vi "Testing Mode.vi"(8 "Filepath":path=path "D:/My Project/2019-2020/Magnetic Mareli UM/MM_UM/Project Setup/data/program seq/Program_280A.bin") -> (4 "Running Model":string)   [LabVIEW 2020]
uses:
  Control Button/Exit.ctl
  Control Button/Start.ctl
  Test  enqueue/AutoTest seq.ctl
  Test  enqueue/Auot Test selection.ctl
  Galobal variable_TI.vi
  Project Setup/Globle Variable/GR_Servo.vi
  <vilib>/Utility/file.llb/Read Delimited Spreadsheet (string).vi
  <vilib>/Utility/file.llb/Write Delimited Spreadsheet (string).vi
panel:
  out "Lc":dbl
  in  "Boolean":bool=TRUE
  in  "String":string
  out "Camera NG":bool
  out "Camera Ok":bool
  out "CO-ORDINATE":T1
  out "Reset":bool
  out "Emergency":bool
  out "Max Load(N)":string
  out "Min Load(N)":string
  in  "Actual Load(N)":string
  out "PPH Max(mm)":string
  out "PPH Min(mm)":string
  out "PPH(mm)":string
  out "Load Cell":dbl format="%0.03f"
  in  "Load Offset":dbl
  out "TFT Code":string
  out "Difus.Code":string
  out "max value":dbl
  out "Difusser Barcode":string
  out "Camera NG_":bool
  out "Camera OK_":bool
  out "Difusser_AI5":bool
  out "Difusser_AI4":bool
  out "Job ID":string
  in  "Graph Reset":bool
  in  "Safety Enb":bool
  in  "LCD Servo Call":bool
  out "Home":bool
  out "Start":bool
  in  "Tab Control":enum32{"Test", "Home call"}(tab)
  in  "test":string[][](table)=[["1", "Light Box Ionization", "Pass"], ["2", "Light box Clamp", "Pass"], ["3", "Difusser Put on Light Box", "Pass"], ["4", "Photo Prism Put On LB", "Test In Progress"], ["5", "LCD Put On Light Box", ""], ["6", "Difusser Checking Position", ""], ["7", "Adesive Tap check Camera", ""], ["8", "LCD Placing Position", ""], ["9", "Camera check Adhesive Taps", ""], ["10", "LCD Display Rotating ", ""], ["11", "Camera Slide Unit", ""], ["12", "LCD Pressing Servo", ""], ["13", "LCD Pressing servo up", ""], ["14", "Camera Unit Rev", ""], ["15", "Fixture Slide Up", ""], ["16", "Light Box Unclamp", ""]]
  in  "Home":string[][](table)
  out "stripped path":path
  in  "Tab":enum32{"Image Display", "Load Graph"}(tab)
  out "2D Picture":picture
  out "Boolean 3":bool
  out "Force Vs Time":dbl[](graph)
  in  "Vacuum bit":bool
  in  "LCD Servo Reset 2":bool
  out "LCD Barcode":string
  out "Date time":string
  in  "NG Counter":string
  in  "OK Counter":string
  out "User Name":string
  out "Error":bool
  in  "Cycle":i32
  in  "Slide Servo Home Call":bool
  out "D-enqueue":T2
  in  "Home Call":bool
  out "DI":bool[](array[boolean])
  in  "Error Message":string
  out "Current Date & Time":timestamp
  out "Cycle Time(Sec)":i32
  in  "Start":T3
  in  "Cycle Start Bit":bool
  in  "vi reference":refnum<vi>
  in  "Reset Ct.":bool
  out "error out":errorcluster
  in  "Tbl Refnum":refnum<vi>
  in  "Image Display":bool
  in  "Exit":T4
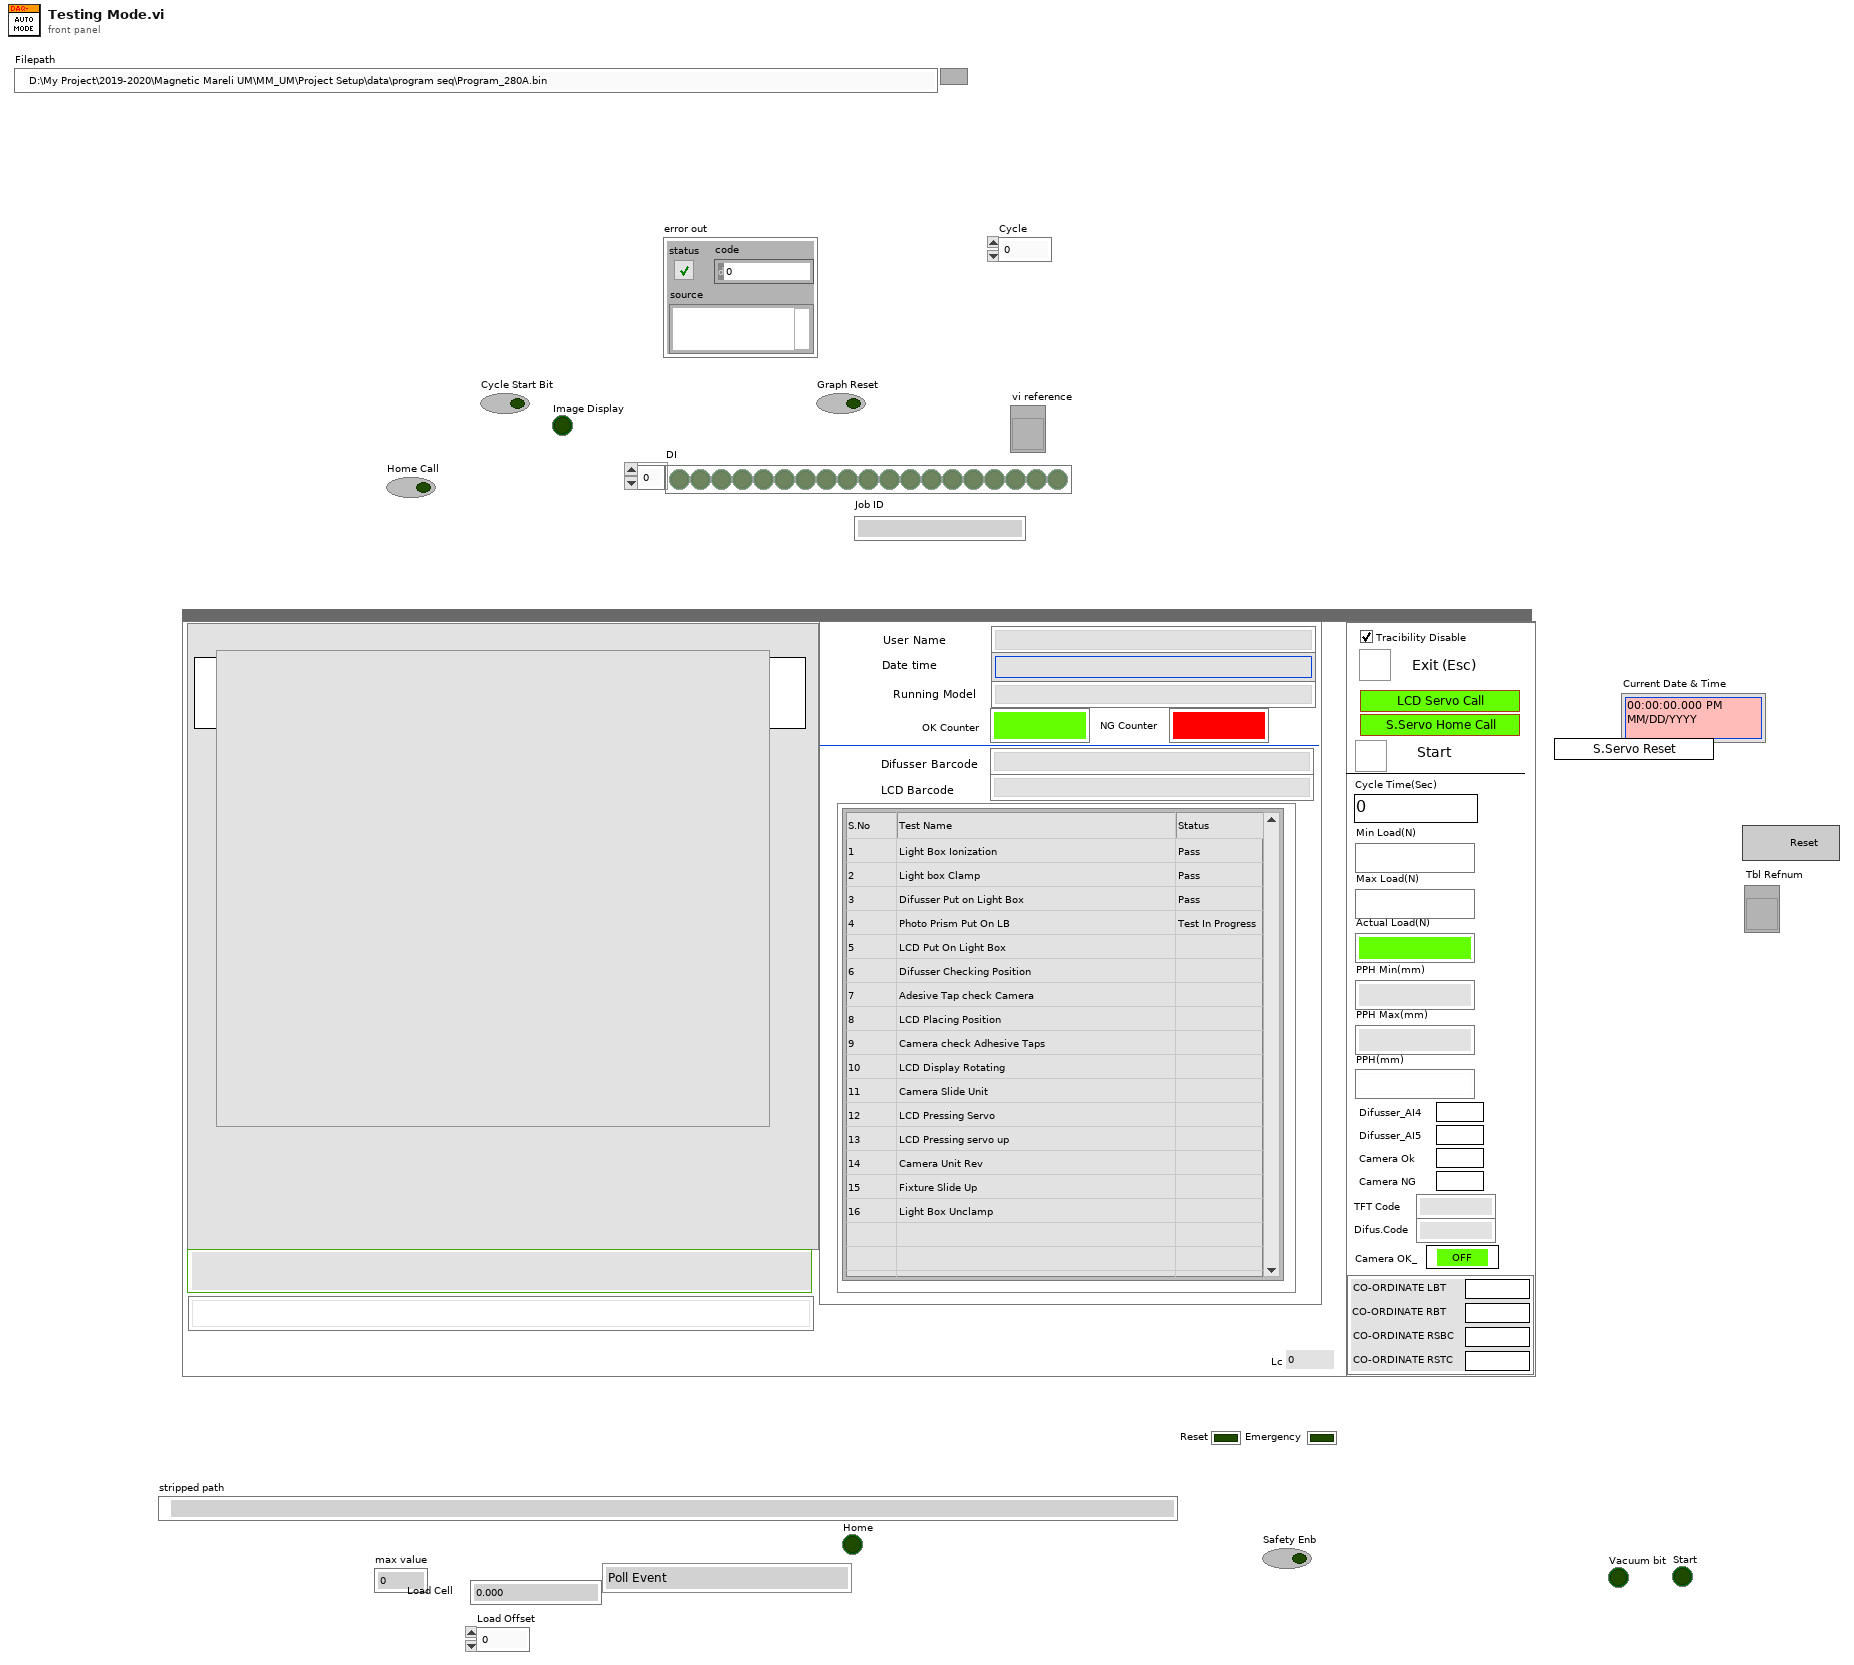
[diagram p1: front panel]
types:
  T1 = cluster{"CO-ORDINATE LBT":string, "CO-ORDINATE RBT":string, "CO-ORDINATE RSBC":string, "CO-ORDINATE RSTC":string}
  T2 = typedef "AutoTest seq.ctl" = enum16{"Poll Event", "Cylender Home ", "Initilization", "Read Barcode", "Slide Servo send Cammand", "Slide Servo Home Call", "LCD Press Servo send Cammand", "LCD Press Servo  Home Call", "Camera Co-ordinate_1", "Home Call", "Result Save", "Exit"}
  T3 = typedef "Start.ctl" = bool
  T4 = typedef "Exit.ctl" = bool
  T5 = typedef "Auot Test selection.ctl" = enum16{"Init", "Enqueue ", "Enqueue N", "Enqueue in stack", "Enqueue in stack N", "Dequeue", "Dequeue N", "Flush", "Release Queue"}
  T6 = cluster{"MaxLoad ":dbl, "Min Load":dbl, "MaxDistance(mm)":dbl, "Min Distance(mm)":dbl, "Load Offset":dbl, "Model":string, "Difusser Code":string, "TFT Code ":string, "LVDT Offset":dbl}
  T7 = cluster{"Item Name":string, "Item Status":bool, "Steps":cluster{"Channel Type":string, "Channels":string, "Wait/Poll (ms)":u32, "Parameter":u8, "STM-Speed":i32, "STM-Degree":u32, "Direction":u8}[]}[]
  T8 = cluster{"No. Fail Coun t":string, "Rework Status Count 0\\1":string, "NA Count Max =3 ":string, "Testesd Count  0/1":string, "Error code":string}
  T9 = enum16{"Height Check Cyl up(P0.23_07)", "Height Check Cyl  Up RS_(AI12_26)", "Height Check Cyl  Dn RS_(AI13_27)", "Height Check Cyl dn(P0.24_08)", "Camera Cyl Rev(P0.26_10)", "Camera Cyl fwd(P0.25_09)", "Height Check Cyl off", "Camera Cyl Rev_RS(AI15_29)", "Camera Cyl off", "Camera Cyl FWD_RS(AI14_28)", "LCD Rotation Dn(P0.28_12)", "LCD Rotation dn proxi(AI17_31)", "LCD Rotation Up(P0.27_11)", "LCD Rotation dn proxi(AI16_30)"}
  T10 = cluster{"Start":bool, "Emergency ":bool, "Reset":bool, "Home":bool, "Safety":bool}
  T11 = cluster{"[0]":string, "[1]":string, "[2]":string, "[3]":string, "[4]":string, "[5]":string, "[6]":string, "[7]":string}
  T12 = cluster{"[0]":string, "[1]":string, "[2]":string, "[3]":string, "[4]":string}
  T13 = cluster{"Emergency":bool, "Air Pressure":bool, "Saftey Sensor":bool, "Slide Servo  fault":bool, "LCD Pressing  Servo  fault":bool, "Reset":bool}
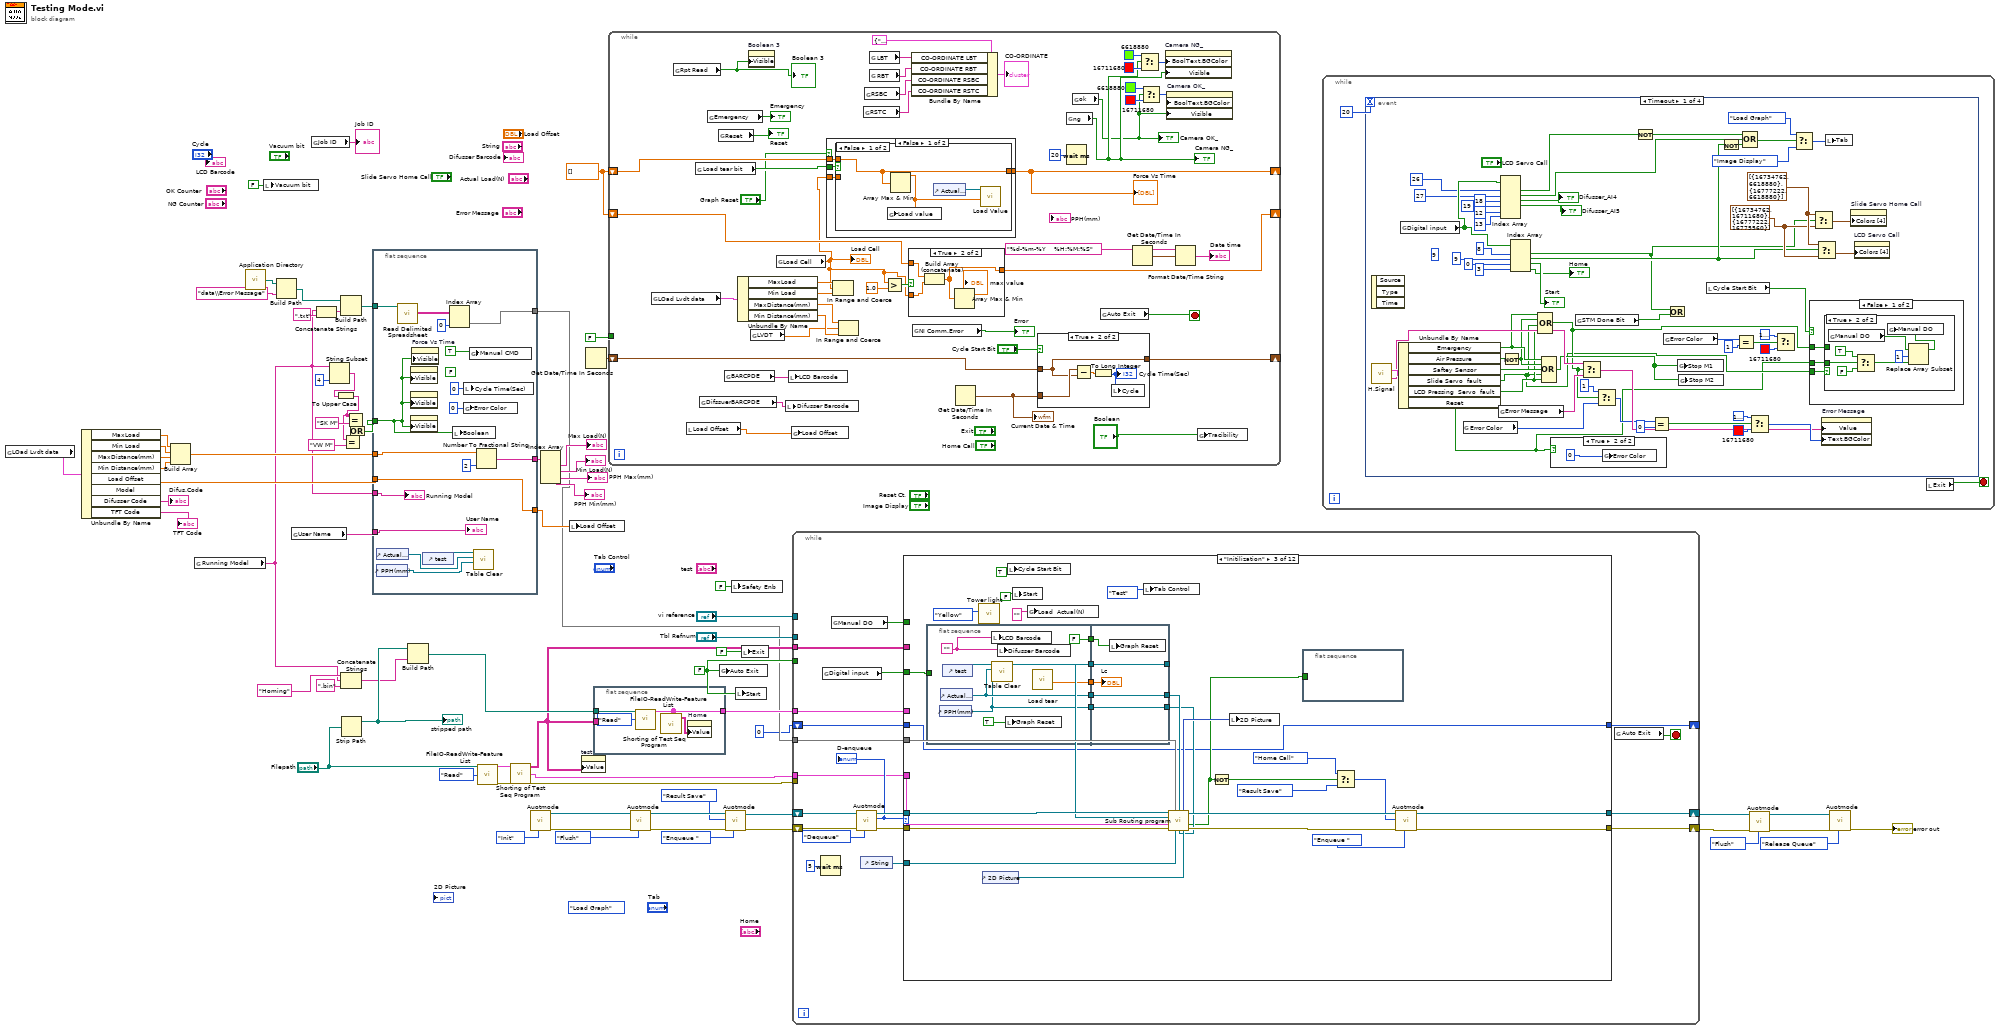
[diagram p0: block diagram]
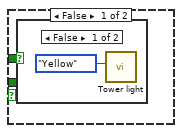
[diagram p3: hidden frame]
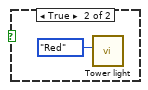
[diagram p4: hidden frame]
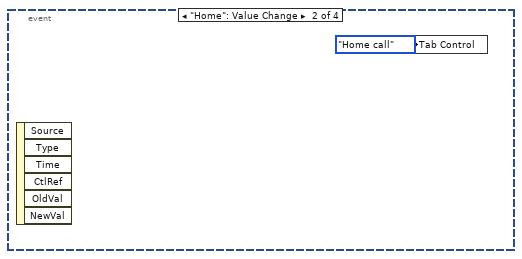
[diagram p6: hidden frame]
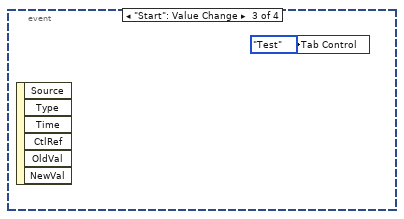
[diagram p7: hidden frame]
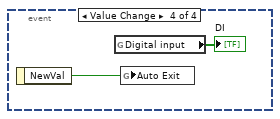
[diagram p8: hidden frame]
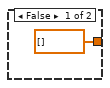
[diagram p9: hidden frame]
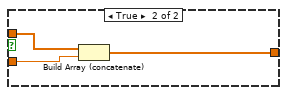
[diagram p10: hidden frame]
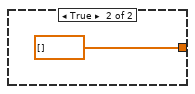
[diagram p11: hidden frame]
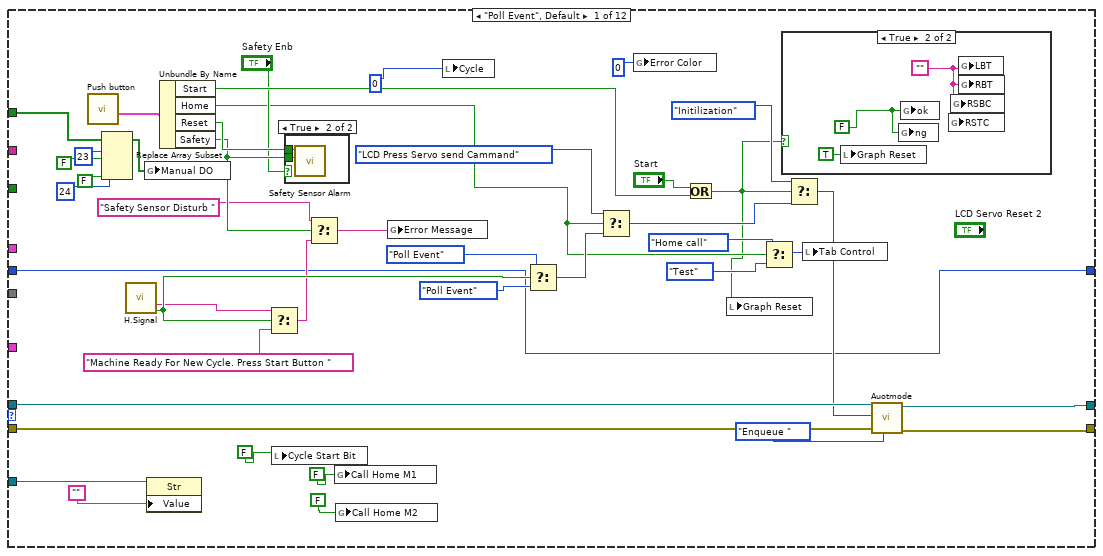
[diagram p13: hidden frame]
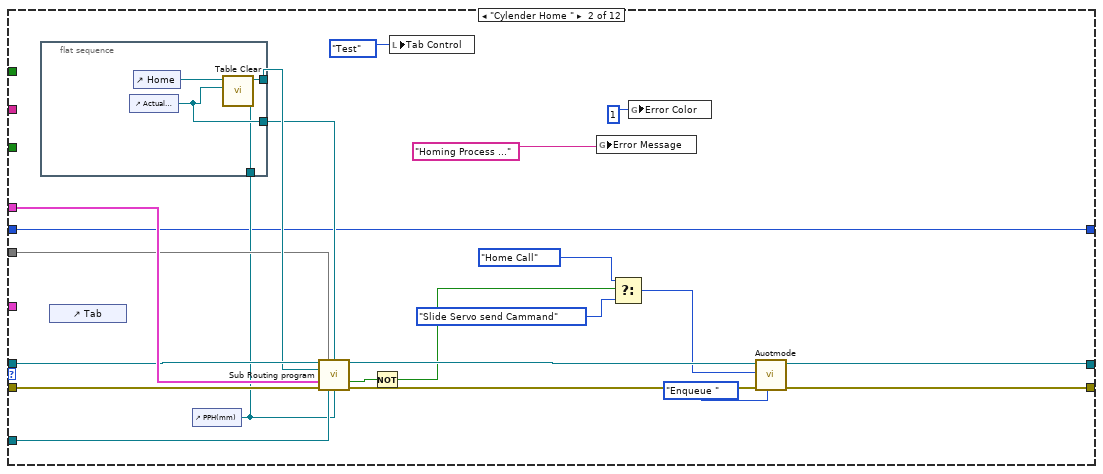
[diagram p16: hidden frame]
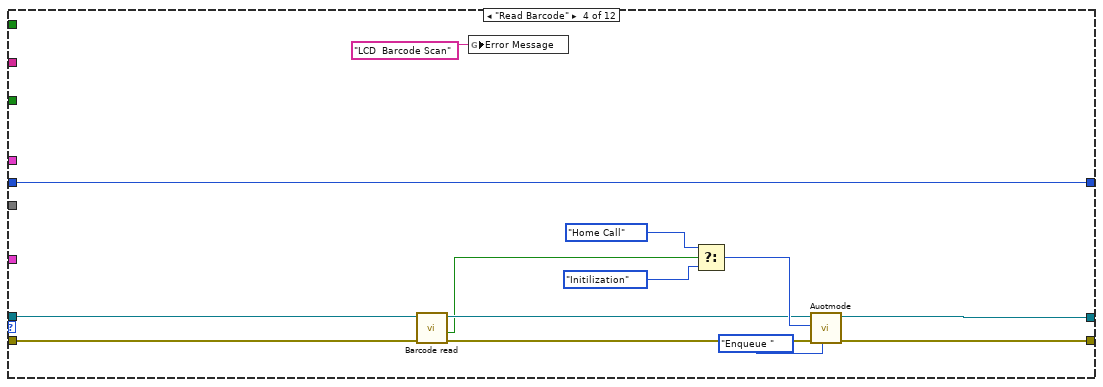
[diagram p17: hidden frame]
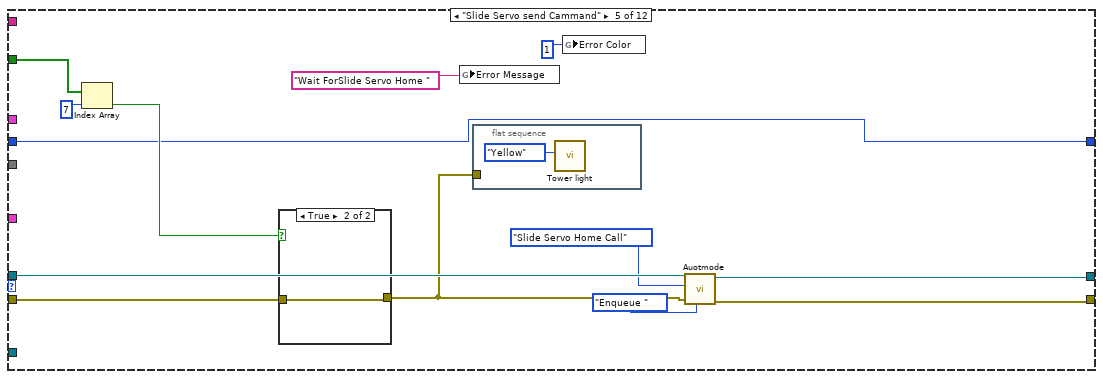
[diagram p18: hidden frame]
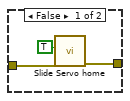
[diagram p19: hidden frame]
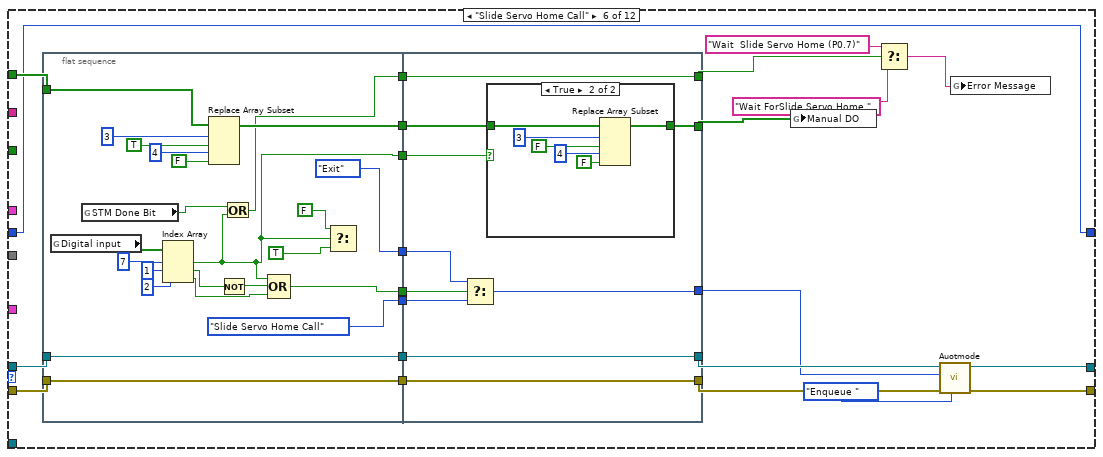
[diagram p20: hidden frame]
diagram:
  (unwired) enum32{"Image Display", "Load Graph"}."Load Graph" ("Tab")
  w29 = dbl[] []
  w47 = FALSE ("Auto Exit")
  n1 = global read "Galobal variable_TI.vi" "LOad Lvdt data"() -> (w28:T6)
  n2 = Unbundle By Name(w28) -> ("MaxLoad"=w27:dbl, "Min Load"=w26:dbl, "MaxDistance(mm)"=w25:dbl, "Min Distance(mm)"=w24:dbl, "Load Offset"=w22:dbl, "Difusser Code"=→"Difus.Code":string, "TFT Code"=→"TFT Code":string)  [unwired: 1 out]
  n3 = Build Array(w27, w26, w25, w24) -> (w23:dbl[])
  n4 = global read "Galobal variable_TI.vi" "Running Model"() -> (w10:string)
  n5 = call <vilib>:"Application Directory.vi"() -> ("Application Directory"=w15:path)
  n6 = local write "Vacuum bit"(FALSE ("Vacuum bit")) -> ()
  n7 = Build Path(base path=w15, name or relative path="data\\Error Message") -> (appended path=w16:path)
  n8 = global read "Galobal variable_TI.vi" "User Name"() -> (w41:string)
  n9 = global read "Galobal variable_TI.vi" "Job ID"() -> (→"Job ID":string)
  n10 = Concatenate Strings(w10, ".txt" ("string")) -> (w13:string)
  n11 = String Subset(string=w10, length (rest)=4 ("length (rest)")) -> (substring=w7:string)  [unwired: 1 in]
  n12 = To Upper Case(1:w7) -> (0:w5:string)
  n13 = Build Path(base path=w16, name or relative path=w13) -> (appended path=w12:path)
  n14 = Concatenate Strings("Homing" ("string"), w10, ".bin" ("string")) -> (w30:string)
  n15 = Strip Path(path="Filepath") -> (stripped path=w38:path)  [unwired: 1 out]
  "stripped path" <- w38
  n16 = Equal?(x=w5, y="VW M") -> (x = y?=w3:bool)
  n17 = Equal?(x=w5, y="SK M") -> (x = y?=w4:bool)
  n18 = Or(x=w3, y=w4) -> (x .or. y?=w2:bool)
  n19 = flat-sequence {
    tunnel: [w86] -> w46
    tunnel: w10 -> [w85]
    tunnel: w41 -> [w84]
    tunnel: [w79] -> w18
    tunnel: w23 -> [w80]
    tunnel: w22 -> [w79]
    tunnel: w12 -> [w77]
    tunnel: [w74] -> w11
    tunnel: w2 -> [w73]
    frame #0 {
      (unwired) FALSE ("LCD Servo Home Call")
      n20 = control-ref of="PPH(mm)"() -> (w81:refnum<vi>)
      n21 = control-ref of="Actual Load(N)"() -> (w82:refnum<vi>)
      n22 = call-poly <vilib>:"Read Delimited Spreadsheet.vi"("file path (dialog if empty)"=w77) -> ("all rows"=w76:string[][])  [unwired: 9 in, 5 out]
      n23 = property on="Min Load(N)" class="Str"("Visible"=w73) -> ()  [unwired: 2 in, 2 out]
      n24 = property on="Max Load(N)" class="Str"("Visible"=w73) -> ()  [unwired: 2 in, 2 out]
      n25 = property on="Actual Load(N)" class="Str"("Visible"=w73) -> ()  [unwired: 2 in, 2 out]
      n26 = property on="Force Vs Time" class="WFGraph (strict)"("Visible"=w73) -> ()  [unwired: 2 in, 2 out]
      n27 = control-ref of="test"() -> (w83:refnum<vi>)
      n28 = Index Array(array=w76, index (col)=0 ("disabled index (col)")) -> (element=w74:string[])  [unwired: 1 in]
      n29 = local write "Boolean"(w73) -> ()
      n30 = global write "GR_Servo.vi" "Error Color"(0 ("Error Color")) -> ()
      n31 = local write "Cycle Time(Sec)"(0 ("Cycle Time(Sec)")) -> ()
      n32 = global write "Galobal variable_TI.vi" "Manual CMD"(TRUE ("Manual CMD")) -> ()
      n33 = call "Table Clear.vi"("Lvdt"=w81, "Load"=w82, "Table (In)"=w83) -> ()  [unwired: 7 in, 2 out]
      n34 = Number To Fractional String(number=w80, precision (6)=i16 2) -> (F-format string=w86:string[])  [unwired: 2 in]
      "User Name" <- w84
      "Running Model" <- w85
    }
  }
  n35 = Build Path(base path=w38, name or relative path=w30) -> (appended path=w37:path)
  n36 = call "FileIO-ReadWrite-FeatureList.vi"("Filepath"="Filepath", "Read/Write"=enum16{"Read", "Write"}."Read") -> ("Feature List (Out)"=w53:T7, "Error Out"=w54:errorcluster)  [unwired: 12 in]
  n37 = call "Shorting of Test Seq Program.vi"("Feature List (Out)"=w53) -> ("Feature Step Enable"=w48:T7, "Feature Name"=w36:string[][])  [unwired: 3 in]
  n38 = call "Auotmode.vi"("Enum Selection"=Auot_Test_selection."Init") -> ("error out"=w66:errorcluster, "queue Out"=w64:refnum<queue>)  [unwired: 7 in, 1 out]
  n39 = Index Array(array=w46) -> (element #1=→"Max Load(N)":string, element #2=→"Min Load(N)":string, element #3=→"PPH Max(mm)":string, element #4=→"PPH Min(mm)":string)  [unwired: 4 in]
  n40 = local write "Load Offset"(w18) -> ()
  n41 = property on="test" class="Tbl (strict)"("Value"=w36) -> ()  [unwired: 2 in, 2 out]
  n42 = Get Date/Time In Seconds() -> (seconds since 1Jan1904=w56:timestamp)
  n43 = flat-sequence {
    tunnel: w37 -> [w92]
    tunnel: w36 -> [_]
    tunnel: [w91] -> w35
    frame #0 {
      n44 = call "FileIO-ReadWrite-FeatureList.vi"("Filepath"=w92, "Read/Write"=enum16{"Read", "Write"}."Read") -> ("Feature List (Out)"=w91:T7)  [unwired: 12 in, 1 out]
      n45 = call "Shorting of Test Seq Program.vi"("Feature List (Out)"=w91) -> ("Feature Name"=w90:string[][])  [unwired: 3 in, 1 out]
      n46 = property on="Home" class="Tbl (strict)"("Value"=w90) -> ()  [unwired: 2 in, 2 out]
    }
  }
  n47 = while {
    shift-right: [w139] -> _
    shift-left: w56 -> [w138]
    tunnel: FALSE ("Servo Stop") -> [_]
    shift-right: [w120] -> _
    shift-left: w29 -> [w122]
    shift-right: [w113] -> _
    shift-left: w29 -> [w115]
    stop <- w136 stop-if-true
    n48 = global read "Galobal variable_TI.vi" "LOad Lvdt data"() -> (w129:T6)
    n49 = global read "Galobal variable_TI.vi" "Rpt Read"() -> (w94:bool)
    "Boolean 3" <- w94
    n50 = local read "Load Offset"() -> (w112:dbl)
    n51 = global read "Galobal variable_TI.vi" "Load tear bit"() -> (w123:bool)
    n52 = global read "Galobal variable_TI.vi" "DifssuerBARCPDE"() -> (w118:string)
    n53 = global read "Galobal variable_TI.vi" "Emergency"() -> (→"Emergency":bool)
    n54 = global read "Galobal variable_TI.vi" "Reset"() -> (→"Reset":bool)
    n55 = global read "Galobal variable_TI.vi" "BARCPDE"() -> (w119:string)
    n56 = Unbundle By Name(w129) -> ("MaxLoad"=w128:dbl, "Min Load"=w127:dbl, "MaxDistance(mm)"=w126:dbl, "Min Distance(mm)"=w125:dbl)
    n57 = property on="Boolean 3" class="Bool (strict)"("Visible"=w94) -> ()  [unwired: 2 in, 2 out]
    n58 = global read "Galobal variable_TI.vi" "LVDT"() -> (w124:dbl)
    n59 = global read "Galobal variable_TI.vi" "Load Cell"() -> (w114:dbl)
    "Load Cell" <- w114
    n60 = local write "Difusser Barcode"(w118) -> ()
    n61 = local write "LCD Barcode"(w119) -> ()
    n62 = global write "Galobal variable_TI.vi" "Load Offset"(w112) -> ()
    n63 = case shown="False" "Graph Reset" {
      tunnel: w123 -> [w148 _]
      tunnel: w114 -> [w147 _]
      tunnel: [w146 dbl[] []] -> w120
      tunnel: w122 -> [w145 _]
      frame False {
        n64 = case shown="False" w148 {
          tunnel: w147 -> [_ w154]
          tunnel: [w151 w152] -> w146
          tunnel: w145 -> [w151 w153]
          frame False {
            n65 = Array Max & Min(array=w151) -> (max value=w149:dbl)  [unwired: 3 out]
            n66 = global write "Galobal variable_TI.vi" "Load value"(w149) -> ()
            n67 = control-ref of="Actual Load(N)"() -> (w150:refnum<vi>)
            n68 = call "Load Value.vi"("Load Cell"=w149, "String in"=w150) -> ()  [unwired: 9 in]
          }
          frame True {
            n69 = Build Array (concatenate)(w153, w154) -> (w152:dbl[])
          }
        }
      }
      frame True {
      }
    }
    "Force Vs Time" <- w120
    n70 = In Range and Coerce(upper limit=w128, x=w114, lower limit=w127) -> ()  [unwired: 2 out]
    n71 = In Range and Coerce(upper limit=w126, x=w124, lower limit=w125) -> ()  [unwired: 2 out]
    n72 = global read "Galobal variable_TI.vi" "RSTC"() -> (w101:string)
    n73 = global read "Galobal variable_TI.vi" "RSBC"() -> (w100:string)
    n74 = global read "Galobal variable_TI.vi" "LBT"() -> (w98:string)
    n75 = global read "Galobal variable_TI.vi" "RBT"() -> (w99:string)
    n76 = Greater?(x=w114, y=1.0) -> (0:w116:bool)
    n77 = case shown="True" w116 {
      tunnel: w115 -> [_ w143]
      tunnel: w114 -> [_ w142]
      tunnel: [dbl[] [] w141] -> w113
      frame False {
      }
      frame True {
        n78 = Build Array (concatenate)(w143, w142) -> (w141:dbl[])
        n79 = Array Max & Min(array=w141) -> (max value=→"max value":dbl)  [unwired: 3 out]
      }
    }
    n80 = Bundle By Name(cluster=T1 {"CO-ORDINATE LBT"="", "CO-ORDINATE RBT"="", "CO-ORDINATE RSBC"="", "CO-ORDINATE RSTC"=""} ("CO-ORDINATE  2"), "CO-ORDINATE LBT"=w98, "CO-ORDINATE RBT"=w99, "CO-ORDINATE RSBC"=w100, "CO-ORDINATE RSTC"=w101) -> (→"CO-ORDINATE":T1)
    n81 = global read "Galobal variable_TI.vi" "NI Comm.Error"() -> (→"Error":bool)
    n82 = Get Date/Time In Seconds() -> (seconds since 1Jan1904=w135:timestamp)
    "Current Date & Time" <- w135
    n83 = case shown="True" "Cycle Start Bit" {
      tunnel: w138 -> [_ w158]
      tunnel: w135 -> [w156 w159]
      tunnel: [w156 w158] -> w139
      frame False {
      }
      frame True {
        n84 = Subtract(x=w159, y=w158) -> (x-y=w160:dbl)
        n85 = To Long Integer(number=w160) -> (32bit integer=w157:i32)
        "Cycle Time(Sec)" <- w157
        n86 = local write "Cycle"(w157) -> ()
      }
    }
    n87 = global read "Galobal variable_TI.vi" "ng"() -> (w103:bool)
    "Camera NG_" <- w103
    n88 = Wait (ms)(milliseconds to wait=u32 20) -> ()  [unwired: 1 out]
    n89 = global read "Galobal variable_TI.vi" "ok"() -> (w102:bool)
    "Camera OK_" <- w102
    n90 = global read "Galobal variable_TI.vi" "Auto Exit"() -> (w136:bool)
    n91 = Get Date/Time In Seconds() -> (seconds since 1Jan1904=w133:timestamp)
    n92 = Select(t=u32 6618880, s=w103, f=u32 16711680) -> (s? t:f=w106:u32)
    n93 = Select(t=u32 6618880, s=w102, f=u32 16711680) -> (s? t:f=w109:u32)
    n94 = property on="Camera NG_" class="Bool (strict)"("BoolText.BGColor"=w106, "Visible"=w103) -> ()  [unwired: 2 in, 2 out]
    n95 = property on="Camera OK_" class="Bool (strict)"("BoolText.BGColor"=w109, "Visible"=w102) -> ()  [unwired: 2 in, 2 out]
    n96 = Format Date/Time String(time format string (%c)="%d-%m-%Y    %H:%M:%S", seconds (now)=w133) -> (date/time string=→"Date time":string)  [unwired: 1 in]
    n97 = global write "Galobal variable_TI.vi" "Tracibility"("Boolean") -> ()
  }
  n98 = call "Auotmode.vi"("Enum Selection"=Auot_Test_selection."Flush", "Error In"=w66, "queue in"=w64) -> ("error out"=w65:errorcluster, "queue Out"=w63:refnum<queue>)  [unwired: 5 in, 1 out]
  n99 = global write "Galobal variable_TI.vi" "Auto Exit"(w47) -> ()
  n100 = call "Auotmode.vi"("Enum Selection"=Auot_Test_selection."Enqueue ", "Error In"=w65, "Enqueue"=AutoTest_seq."Result Save", "queue in"=w63) -> ("error out"=w70:errorcluster, "queue Out"=w51:refnum<queue>)  [unwired: 4 in, 1 out]
  n101 = local write "Safety Enb"(FALSE ("Safety Enb")) -> ()
  n102 = local write "Start"(w47) -> ()
  n103 = local write "Exit"(T4 FALSE ("Exit")) -> ()
  n104 = while {
    tunnel: "vi reference" -> [_]
    tunnel: "Tbl Refnum" -> [_]
    tunnel: w48 -> [w172]
    tunnel: w54 -> [_]
    tunnel: w11 -> [w173]
    shift-right: [w176] -> w57
    shift-left: w51 -> [w169]
    shift-right: [w168] -> w50
    shift-left: w70 -> [w178]
    tunnel: w47 -> [_]
    tunnel: w36 -> [w167]
    tunnel: w35 -> [w164]
    shift-right: [w161] -> _
    shift-left: 0 -> [w162]
    stop <- w171 stop-if-true
    n105 = Wait (ms)(milliseconds to wait=u32 5) -> ()  [unwired: 1 out]
    n106 = global read "Galobal variable_TI.vi" "Digital input"() -> (w166:bool[])
    n107 = global read "Galobal variable_TI.vi" "Manual DO"() -> (w165:bool[])
    n108 = call "Auotmode.vi"("Enum Selection"=Auot_Test_selection."Dequeue", "Error In"=w178, "queue in"=w169) -> ("error out"=w175:errorcluster, "D-enqueue"=w174:T2, "queue Out"=w177:refnum<queue>)  [unwired: 5 in]
    "D-enqueue" <- w174
    n109 = control-ref of="String"() -> (w163:refnum<vi>)
    n110 = case shown="\"Initilization\"" w174 {
      tunnel: w177 -> [w222 w245 w284 w311 w320 w349 w404 w421 w439 w453 w507 w577]
      tunnel: [w220 w249 w279 w304 w323 w350 w402 w420 w439 w452 w506 w578] -> w176
      tunnel: w175 -> [w221 w243 w283 w310 w321 w348 w406 w419 w438 w451 w505 w580]
      tunnel: [w219 w248 w278 w302 w322 w351 w401 w418 w438 w450 w504 w580] -> w168
      tunnel: w172 -> [_ _ w285 _ _ _ _ _ _ _ _ _]
      tunnel: w173 -> [_ w240 w275 _ _ _ _ _ _ _ _ _]
      tunnel: w167 -> [_ _ _ _ _ _ _ _ _ _ _ _]
      tunnel: w166 -> [_ _ w271 _ w317 _ w400 _ _ w447 _ _]
      tunnel: w165 -> [w186 _ _ _ _ w336 _ w427 _ _ _ _]
      tunnel: w164 -> [_ w246 _ _ _ _ _ _ _ _ _ _]
      tunnel: w163 -> [w203 w234 w267 _ _ _ _ _ _ _ _ _]
      tunnel: w162 -> [w180 w228 w255 w299 w312 w330 w393 w412 w437 w441 w502 w560]
      tunnel: [w180 w228 w255 w299 w312 w330 w393 w412 w437 w440 w501 w560] -> w161
      frame "Poll Event", Default {
        n111 = call "Push button.vi"() -> ("Push Button"=w205:T10)  [unwired: 11 in]
        n112 = Replace Array Subset(array=w186, new element #1=FALSE ("new element/subarray"), index #1=23 ("index"), new element #2=FALSE ("new element/subarray"), index #2=24 ("index")) -> (w181:bool[])
        n113 = call "H.Signal.vi"() -> ("Error Message"=w187:string, "Bool_H Sig"=w199:bool)  [unwired: 10 in, 4 out]
        n114 = global write "Galobal variable_TI.vi" "Manual DO"(w181) -> ()
        n115 = property class="Str"(reference=w203, "Value"="") -> ()  [unwired: 1 in, 2 out]
        n116 = Unbundle By Name(w205) -> ("Start"=w204:bool, "Home"=w190:bool, "Reset"=w201:bool, "Safety"=w198:bool)
        n117 = Select(t=w187, s=w199, f="Machine Ready For New Cycle. Press Start Button ") -> (s? t:f=w196:string)
        n118 = local write "Cycle Start Bit"(FALSE ("Cycle Start Bit")) -> ()
        n119 = case shown="True" "Safety Enb" {
          tunnel: w201 -> [_ w227]
          tunnel: w198 -> [_ w226]
          frame False {
          }
          frame True {
            n120 = call "Safety Sensor Alarm.vi"("Safety"=w226, "Reset"=w227) -> ()  [unwired: 10 in]
          }
        }
        n121 = Select(t="Safety Sensor Disturb " ("f"), s=w198, f=w196) -> (s? t:f=w195:string)
        n122 = global write "Galobal variable_TI.vi" "Call Home M1"(FALSE ("Call Home M1")) -> ()
        n123 = global write "Galobal variable_TI.vi" "Call Home M2"(FALSE ("Call Home M1")) -> ()
        n124 = global write "GR_Servo.vi" "Error Message"(w195) -> ()
        n125 = local write "Cycle"(0 ("Cycle")) -> ()
        n126 = Select(t=AutoTest_seq."Poll Event" ("Enqueue"), s=w199, f=AutoTest_seq."Poll Event") -> (s? t:f=w210:T2)
        n127 = Select(t=AutoTest_seq."LCD Press Servo send Cammand" ("Enqueue"), s=w190, f=w210) -> (s? t:f=w213:T2)
        n128 = global write "GR_Servo.vi" "Error Color"(0 ("Error Color")) -> ()
        n129 = Or(x="Start", y=w204) -> (x .or. y?=w188:T3)
        n130 = local write "Graph Reset"(w188) -> ()
        n131 = Select(t=enum32{"Test", "Home call"}."Home call" ("Tab Control"), s=w190, f=enum32{"Test", "Home call"}."Test" ("Tab Control")) -> (s? t:f=w192:enum32{"Test", "Home call"})
        n132 = case shown="True" w188 {
          frame False {
          }
          frame True {
            w223 = ""
            w224 = FALSE
            n133 = local write "Graph Reset"(TRUE ("Boolean")) -> ()
            n134 = global write "Galobal variable_TI.vi" "ng"(w224) -> ()
            n135 = global write "Galobal variable_TI.vi" "ok"(w224) -> ()
            n136 = global write "Galobal variable_TI.vi" "RSTC"(w223) -> ()
            n137 = global write "Galobal variable_TI.vi" "RSBC"(w223) -> ()
            n138 = global write "Galobal variable_TI.vi" "LBT"(w223) -> ()
            n139 = global write "Galobal variable_TI.vi" "RBT"(w223) -> ()
          }
        }
        n140 = Select(t=AutoTest_seq."Initilization" ("Enqueue"), s=w188, f=w213) -> (s? t:f=w212:T2)
        n141 = local write "Tab Control"(w192) -> ()
        n142 = call "Auotmode.vi"("Enum Selection"=Auot_Test_selection."Enqueue ", "Error In"=w221, "Enqueue"=w212, "queue in"=w222) -> ("error out"=w219:errorcluster, "queue Out"=w220:refnum<queue>)  [unwired: 4 in, 1 out]
      }
      frame "Cylender Home " {
        n143 = flat-sequence {
          tunnel: [w253] -> w241
          tunnel: [w251] -> w233
          tunnel: w232 -> [w250]
          frame #0 {
            n144 = control-ref of="Actual Load(N)"() -> (w251:refnum<vi>)
            n145 = control-ref of="Home"() -> (w252:refnum<vi>)
            n146 = call "Table Clear.vi"("Lvdt"=w250, "Load"=w251, "Table (In)"=w252) -> ("Table (Out)"=w253:refnum<vi>)  [unwired: 7 in, 1 out]
          }
        }
        n147 = control-ref of="Tab"() -> ()  [unwired: 1 out]
        n148 = control-ref of="PPH(mm)"() -> (w232:refnum<vi>)
        n149 = call "Sub Routing program.vi"("queue Out in"=w245, "FeedBack Channel"=w240, "Load"=w233, "reference in"=w241, "Feature Step Enable"=w246, "error in (no error)"=w243, "Str Refnum"=w234, "Lvdt"=w232) -> ("Queue out"=w244:refnum<queue>, "Result"=w237:bool, "error out"=w242:errorcluster)  [unwired: 3 in, 2 out]
        n150 = Not(x=w237) -> (.not. x?=w236:bool)
        n151 = local write "Tab Control"(enum32{"Test", "Home call"}."Test" ("Tab Control")) -> ()
        n152 = global write "GR_Servo.vi" "Error Message"("Homing Process ...") -> ()
        n153 = Select(t=AutoTest_seq."Home Call" ("Enqueue"), s=w236, f=AutoTest_seq."Slide Servo send Cammand" ("Enqueue")) -> (s? t:f=w235:T2)
        n154 = global write "GR_Servo.vi" "Error Color"(1 ("Error Color")) -> ()
        n155 = call "Auotmode.vi"("Enum Selection"=Auot_Test_selection."Enqueue ", "Error In"=w242, "Enqueue"=w235, "queue in"=w244) -> ("error out"=w248:errorcluster, "queue Out"=w249:refnum<queue>)  [unwired: 4 in, 1 out]
      }
      frame "Initilization" {
        n156 = flat-sequence {
          tunnel: w271 -> [_]
          tunnel: [w292] -> w260
          tunnel: [w291] -> w259
          tunnel: [w290] -> w258
          tunnel: [FALSE ("Graph Reset")] -> w257
          tunnel: [w286] -> w254
          tunnel: [w296] -> w262
          tunnel: [w297] -> w263
          tunnel: [w298] -> w270
          tunnel: w260 -> [w298]
          tunnel: w259 -> [w297]
          tunnel: w258 -> [w296]
          tunnel: w257 -> [w295]
          tunnel: w254 -> [w294]
          frame #0 {
            w289 = ""
            n157 = control-ref of="PPH(mm)"() -> (w290:refnum<vi>)
            n158 = control-ref of="Actual Load(N)"() -> (w291:refnum<vi>)
            n159 = control-ref of="test"() -> (w293:refnum<vi>)
            n160 = local write "LCD Barcode"(w289) -> ()
            n161 = call "Table Clear.vi"("Lvdt"=w290, "Load"=w291, "Table (In)"=w293) -> ("Table (Out)"=w292:refnum<vi>)  [unwired: 7 in, 1 out]
            n162 = local write "Difusser Barcode"(w289) -> ()
            n163 = local write "Graph Reset"(TRUE ("Boolean")) -> ()
            n164 = call "Load tear.vi"() -> ("Load Cell"=w286:dbl)  [unwired: 11 in]
          }
          frame #1 {
            n165 = local write "Graph Reset"(w295) -> ()
            "Lc" <- w294
          }
        }
        n166 = call "Tower light.vi"("Enum"=enum16{"Green", "Red", "Yellow"}."Yellow") -> ()  [unwired: 11 in]
        n167 = control-ref of="2D Picture"() -> (w266:refnum<vi>)
        n168 = local write "Cycle Start Bit"(TRUE ("Cycle Start Bit")) -> ()
        n169 = local write "Start"(T3 FALSE ("Start")) -> ()
        n170 = global write "Galobal variable_TI.vi" "Load  Actual(N)"("" ("Load  Actual(N)")) -> ()
        n171 = local write "Tab Control"(enum32{"Test", "Home call"}."Test" ("Tab Control")) -> ()
        n172 = call "Sub Routing program.vi"("queue Out in"=w284, "FeedBack Channel"=w275, "Load"=w263, "reference in"=w270, "Feature Step Enable"=w285, "error in (no error)"=w283, "Str Refnum"=w267, "Lvdt"=w262, "Pict Refnum"=w266) -> ("2D Picture"=w268:picture, "Queue out"=w281:refnum<queue>, "Result"=w261:bool, "error out"=w280:errorcluster)  [unwired: 2 in, 1 out]
        n173 = Not(x=w261) -> (.not. x?=w269:bool)
        n174 = local write "2D Picture"(w268) -> ()
        n175 = flat-sequence {
          tunnel: w261 -> [_]
          frame #0 {
          }
        }
        n176 = Select(t=AutoTest_seq."Home Call" ("Enqueue"), s=w269, f=AutoTest_seq."Result Save" ("Enqueue")) -> (s? t:f=w272:T2)
        n177 = call "Auotmode.vi"("Enum Selection"=Auot_Test_selection."Enqueue ", "Error In"=w280, "Enqueue"=w272, "queue in"=w281) -> ("error out"=w278:errorcluster, "queue Out"=w279:refnum<queue>)  [unwired: 4 in, 1 out]
      }
      frame "Read Barcode" {
        n178 = call "Barcode read.vi"("error in"=w310, "queue in"=w311) -> ("error out"=w303:errorcluster, "exit"=w300:bool, "queue Out 2"=w305:refnum<queue>)  [unwired: 6 in, 1 out]
        n179 = global write "GR_Servo.vi" "Error Message"("LCD  Barcode Scan") -> ()
        n180 = Select(t=AutoTest_seq."Home Call" ("Enqueue"), s=w300, f=AutoTest_seq."Initilization" ("Enqueue")) -> (s? t:f=w309:T2)
        n181 = call "Auotmode.vi"("Enum Selection"=Auot_Test_selection."Enqueue ", "Error In"=w303, "Enqueue"=w309, "queue in"=w305) -> ("error out"=w302:errorcluster, "queue Out"=w304:refnum<queue>)  [unwired: 4 in, 1 out]
      }
      frame "Slide Servo send Cammand" {
        n182 = Index Array(array=w317, index=7) -> (element=w316:bool)
        n183 = case shown="True" w316 {
          tunnel: w321 -> [w327 w328]
          tunnel: [w325 w328] -> w318
          frame False {
            n184 = call "Slide Servo home.vi"("error in"=w327, "NewVal"=TRUE) -> ("error out"=w325:errorcluster)  [unwired: 9 in]
          }
          frame True {
          }
        }
        n185 = global write "GR_Servo.vi" "Error Message"("Wait ForSlide Servo Home ") -> ()
        n186 = flat-sequence {
          tunnel: w318 -> [_]
          frame #0 {
            n187 = call "Tower light.vi"("Enum"=enum16{"Green", "Red", "Yellow"}."Yellow") -> ()  [unwired: 11 in]
          }
        }
        n188 = global write "GR_Servo.vi" "Error Color"(1 ("Error Color")) -> ()
        n189 = call "Auotmode.vi"("Enum Selection"=Auot_Test_selection."Enqueue ", "Error In"=w318, "Enqueue"=AutoTest_seq."Slide Servo Home Call", "queue in"=w320) -> ("error out"=w322:errorcluster, "queue Out"=w323:refnum<queue>)  [unwired: 4 in, 1 out]
      }
      frame "Slide Servo Home Call" {
        n190 = flat-sequence {
          tunnel: w349 -> [w371]
          tunnel: w348 -> [w370]
          tunnel: [w371] -> w345
          tunnel: [w370] -> w344
          tunnel: [AutoTest_seq."Exit" ("Enqueue")] -> w343
          tunnel: [AutoTest_seq."Slide Servo Home Call" ("Enqueue")] -> w342
          tunnel: [w358] -> w341
          tunnel: [w362] -> w339
          tunnel: [w357] -> w337
          tunnel: w336 -> [w356]
          tunnel: [w353] -> w335
          tunnel: [w384] -> w346
          tunnel: [w385] -> w347
          tunnel: w345 -> [w385]
          tunnel: w344 -> [w384]
          tunnel: w343 -> [w383]
          tunnel: w342 -> [w382]
          tunnel: w341 -> [w380]
          tunnel: [w381] -> w340
          tunnel: w339 -> [w379]
          tunnel: [w378] -> w338
          tunnel: w337 -> [w377]
          tunnel: [w376] -> w334
          tunnel: w335 -> [w376]
          frame #0 {
            n191 = global read "Galobal variable_TI.vi" "Digital input"() -> (w367:bool[])
            n192 = global read "Galobal variable_TI.vi" "STM Done Bit"() -> (w374:bool)
            n193 = Index Array(array=w367, index #1=7 ("index"), index #2=1 ("index"), index #3=2 ("index")) -> (element #1=w357:bool, element #2=w360:bool, element #3=w354:bool)
            n194 = Replace Array Subset(array=w356, new element #1=TRUE ("new element/subarray"), index #1=3 ("index"), new element #2=FALSE ("new element/subarray"), index #2=4 ("index")) -> (w362:bool[])
            n195 = Not(x=w360) -> (.not. x?=w359:bool)
            n196 = Or(x=w374, y=w357) -> (x .or. y?=w353:bool)
            n197 = Compound Arithmetic op=OR(w357, w359, w354) -> (w358:bool)
            n198 = Select(t=FALSE, s=w357, f=TRUE) -> ()  [unwired: 1 out]
          }
          frame #1 {
            n199 = Select(t=w383, s=w380, f=w382) -> (s? t:f=w381:T2)
            n200 = case shown="True" w377 {
              tunnel: w379 -> [w386 w388]
              tunnel: [w386 w387] -> w378
              frame False {
              }
              frame True {
                n201 = Replace Array Subset(array=w388, new element #1=FALSE ("new element/subarray"), index #1=3 ("index"), new element #2=FALSE ("new element/subarray"), index #2=4 ("index")) -> (w387:bool[])
              }
            }
          }
        }
        n202 = global write "Galobal variable_TI.vi" "Manual DO"(w338) -> ()
        n203 = Select(t="Wait  Slide Servo Home (P0.7)", s=w334, f="Wait ForSlide Servo Home ") -> (s? t:f=w331:string)
        n204 = call "Auotmode.vi"("Enum Selection"=Auot_Test_selection."Enqueue ", "Error In"=w346, "Enqueue"=w340, "queue in"=w347) -> ("error out"=w351:errorcluster, "queue Out"=w350:refnum<queue>)  [unwired: 4 in, 1 out]
        n205 = global write "GR_Servo.vi" "Error Message"(w331) -> ()
      }
      frame "LCD Press Servo send Cammand" {
        n206 = Index Array(array=w400, index=9) -> (element=w396:bool)
        n207 = case shown="True" w396 {
          tunnel: w406 -> [w410 w411]
          tunnel: [w408 w411] -> w403
          frame False {
            n208 = call "LCD Servo Home Call.vi"("error in"=w410, "Enable(T)/Dissable"=TRUE) -> ("error out"=w408:errorcluster)  [unwired: 9 in]
          }
          frame True {
          }
        }
        n209 = global write "GR_Servo.vi" "Error Color"(1 ("Error Color")) -> ()
        n210 = Select(t="Wait For LCD Pressing Servo Home ", s=w396, f="Wait  Slide Servo Home (P0.9)") -> (s? t:f=w397:string)
        n211 = global write "GR_Servo.vi" "Error Message"(w397) -> ()
        n212 = call "Auotmode.vi"("Enum Selection"=Auot_Test_selection."Enqueue ", "Error In"=w403, "Enqueue"=AutoTest_seq."LCD Press Servo  Home Call", "queue in"=w404) -> ("error out"=w401:errorcluster, "queue Out"=w402:refnum<queue>)  [unwired: 4 in, 1 out]
      }
      frame "LCD Press Servo  Home Call" {
        n213 = global read "Galobal variable_TI.vi" "Digital input"() -> (w428:bool[])
        n214 = Index Array(array=w428, index #1=9 ("index"), index #2=2 ("index")) -> (element #1=w422:bool, element #2=w416:bool)
        n215 = case shown="False" w422 {
          tunnel: [w430 w432] -> w426
          tunnel: w427 -> [w430 w431]
          frame False {
          }
          frame True {
            n216 = Replace Array Subset(array=w431, new element #1=FALSE ("new element/subarray"), index #1=3 ("index"), new element #2=FALSE ("new element/subarray"), index #2=4 ("index")) -> (w432:bool[])
          }
        }
        n217 = global write "Galobal variable_TI.vi" "Manual DO"(w426) -> ()
        n218 = Select(t=AutoTest_seq."Cylender Home " ("Enqueue"), s=w422, f=AutoTest_seq."LCD Press Servo  Home Call" ("Enqueue")) -> (s? t:f=w414:T2)
        n219 = Select(t=AutoTest_seq."Home Call" ("Enqueue"), s=w416, f=w414) -> (s? t:f=w413:T2)
        n220 = call "Auotmode.vi"("Enum Selection"=Auot_Test_selection."Enqueue ", "Error In"=w419, "Enqueue"=w413, "queue in"=w421) -> ("error out"=w418:errorcluster, "queue Out"=w420:refnum<queue>)  [unwired: 4 in, 1 out]
      }
      frame "Camera Co-ordinate_1" {
      }
      frame "Home Call" {
        n221 = Index Array(array=w447, index #1=3 ("index"), index #2=9 ("index")) -> (element #1=w446:bool, element #2=w443:bool)
        n222 = case shown="True" w446 {
          tunnel: [w462 w475] -> w445
          tunnel: enum16{"Green", "Red", "Yellow"}."Red" ("Enum") -> [w466 _]
          tunnel: w443 -> [w463 _]
          tunnel: w441 -> [w459 w473]
          tunnel: [w459 w472] -> w440
          frame False {
            n223 = global read "GR_Servo.vi" "Error Message"() -> (w458:string)
            n224 = call "Tower light.vi"("Enum"=w466) -> ()  [unwired: 11 in]
            n225 = Not(x=w463) -> (.not. x?=w461:bool)
            n226 = Concatenate Strings(w458, "" ("string"), "Press Home Push Button") -> (w457:string)
            n227 = case shown="True" w461 {
              frame False {
              }
              frame True {
                n228 = global read "Galobal variable_TI.vi" "Running Model"() -> (w471:string)
                n229 = call "Working Shift Change(A-B &C).vi"() -> ("Shift Change"=w470:string)  [unwired: 9 in]
                n230 = call "Sub_ shift data reset.vi"("File Name"="OK Counter.txt", "Shift"=w470, "Model"=w471) -> ("Serial no"=w467:string)  [unwired: 6 in, 1 out]
                n231 = property on="NG Counter" class="Str"("Value"=w467, "Text.BGColor"=u32 16711680 ("Color Box")) -> ()  [unwired: 2 in, 2 out]
              }
            }
            n232 = Select(t=AutoTest_seq."LCD Press Servo send Cammand" ("Enqueue"), s=w461, f=AutoTest_seq."Home Call") -> (s? t:f=w462:T2)
            n233 = global write "GR_Servo.vi" "Error Color"(1 ("Error Color")) -> ()
            n234 = global write "GR_Servo.vi" "Error Message"(w457) -> ()
          }
          frame True {
            n235 = flat-sequence {
              tunnel: [AutoTest_seq."LCD Press Servo send Cammand" ("Enqueue")] -> w474
              tunnel: [w499] -> w475
              tunnel: w474 -> [w499]
              frame #0 {
                w493 = FALSE ("Emergency")
                n236 = global read "Galobal variable_TI.vi" "Running Model"() -> (w498:string)
                n237 = global read "Galobal variable_TI.vi" "Shift  Change"() -> (w492:string)
                n238 = global write "Galobal variable_TI.vi" "Emergency"(w493) -> ()
                n239 = global write "Galobal variable_TI.vi" "Reset"(w493) -> ()
                n240 = call "Sub_ shift data reset.vi"("File Name"="OK Counter.txt", "Shift"=w492, "Model"=w498) -> ("Serial no"=w496:string)  [unwired: 6 in, 1 out]
                n241 = property on="NG Counter" class="Str"("Value"=w496, "Text.BGColor"=u32 16711680 ("Color Box")) -> ()  [unwired: 2 in, 2 out]
              }
              frame #1 {
                n242 = flat-sequence {
                  frame #0 {
                    n243 = call "Tower light.vi"("Enum"=enum16{"Green", "Red", "Yellow"}."Yellow") -> ()  [unwired: 11 in]
                  }
                }
              }
            }
            n244 = stacked-sequence {
              seq-local: [w477 _ _] -> [_ _ w491]
              tunnel: w473 -> [w478 _ _]
              tunnel: [_ _ w491] -> w472
              frame #0 {
                n245 = case shown="True" TRUE {
                  tunnel: w478 -> [w479 w483]
                  tunnel: [w479 w482] -> w477
                  frame False {
                  }
                  frame True {
                    n246 = Increment(x=w483) -> (x+1=w482:i32)
                    n247 = Number To Decimal String(number=w482) -> (decimal integer string=w484:string)  [unwired: 1 in]
                    n248 = Bundle By Name(cluster=T8 {"No. Fail Coun t"="", "Rework Status Count 0\\1"="", "NA Count Max =3 "="", "Testesd Count  0/1"="", "Error code"=""} ("Count For Rework"), "No. Fail Coun t"=w484, "Rework Status Count 0\\1"="1" ("Rework Status Count 0\\1"), "NA Count Max =3"="0", "Testesd Count  0/1"="0") -> (w481:T8)
                    n249 = call "Rework Count.vi"("Read /Write"=enum16{"Write", "Read"}."Write", "Count For Rework"=w481) -> ()  [unwired: 8 in, 2 out]
                  }
                }
              }
              frame #1 {
                n250 = Wait (ms)(milliseconds to wait=u32 300) -> ()  [unwired: 1 out]
              }
              frame #2 {
                n251 = global write "Galobal variable_TI.vi" "Rpt Write"(TRUE ("Rpt Write")) -> ()
              }
            }
          }
        }
        n252 = local write "Tab Control"(enum32{"Test", "Home call"}."Home call" ("Tab Control")) -> ()
        n253 = call "Auotmode.vi"("Enum Selection"=Auot_Test_selection."Enqueue ", "Error In"=w451, "Enqueue"=w445, "queue in"=w453) -> ("error out"=w450:errorcluster, "queue Out"=w452:refnum<queue>)  [unwired: 4 in, 1 out]
      }
      frame "Result Save" {
        n254 = stacked-sequence {
          frame #0 {
            (unwired) FALSE ("Pokayoka Status")
            n255 = global read "Galobal variable_TI.vi" "Shift  Change"() -> (w524:string)
            n256 = global read "Galobal variable_TI.vi" "Running Model"() -> (w529:string)
            n257 = global write "Galobal variable_TI.vi" "Rpt Write"(TRUE ("Rpt Write")) -> ()
            n258 = call "Sub_ shift data reset.vi"("File Name"="OK Counter.txt", "Shift"=w524, "Model"=w529) -> ("Serial no"=w526:string)  [unwired: 6 in, 1 out]
            n259 = property on="OK Counter" class="Str"("Value"=w526, "Text.BGColor"=u32 6618880 ("Color Box")) -> ()  [unwired: 2 in, 2 out]
          }
          frame #1 {
            n260 = call "Tower light.vi"("Enum"=enum16{"Green", "Red", "Yellow"}."Green") -> ()  [unwired: 11 in]
          }
          frame #2 {
            n261 = local read "Min Load(N)"() -> (w554:string)
            n262 = local read "Max Load(N)"() -> (w553:string)
            n263 = global read "Galobal variable_TI.vi" "DifssuerBARCPDE"() -> (w532:string)
            n264 = local read "Actual Load(N)"() -> (w552:string)
            n265 = global read "Galobal variable_TI.vi" "Load Status"() -> (w551:string)
            n266 = global read "Galobal variable_TI.vi" "LVDT Status"() -> (w547:string)
            n267 = local read "PPH Min(mm)"() -> (w550:string)
            n268 = local read "PPH Max(mm)"() -> (w549:string)
            n269 = global read "Galobal variable_TI.vi" "BARCPDE"() -> (w533:string)
            n270 = local read "PPH(mm)"() -> (w546:string)
            n271 = global read "Galobal variable_TI.vi" "Running Model"() -> (w557:string)
            n272 = Build Array(w554, w553, w552, w551, w550, w549, w546, w547) -> (w548:string[])
            n273 = local read "Date time"() -> (w559:string)
            n274 = global read "Galobal variable_TI.vi" "User Name"() -> (w558:string)
            n275 = Array To Cluster(array=w548) -> (cluster=w545:T11)
            n276 = local read "test"() -> (w534:string[][])
            n277 = Build Array(w559, w558, w557, w533, w532) -> (w556:string[])
            n278 = Array To Cluster(array=w556) -> (cluster=w555:T12)
            n279 = call <vilib>:"Application Directory.vi"() -> ("Application Directory"=w543:path)
            n280 = call "Report Raw Data.vi"("Data"=w555, "Sensor Data"=w545, "test"=w534) -> ("Machine Status"=w531:bool, "Data"=w537:string[], "Header"=w540:string[])  [unwired: 6 in]
            n281 = global write "Galobal variable_TI.vi" "Pokayoka Status"(w531) -> ()
            n282 = Build Path(base path=w543, name or relative path="data\\Report") -> (appended path=w544:path)
            n283 = call "Header Create.vi"("Report Header"=w540, "File Name"="Test Report", "path File"=w544) -> ("error out"=w538:errorcluster, "dup path"=w539:path)  [unwired: 7 in]
            n284 = call-poly <vilib>:"Write Delimited Spreadsheet.vi"("file path (dialog if empty)"=w539, "1D data"=w537, "append to file? (new file:F)"=TRUE ("append to file? (F)"), "error in (no error)"=w538, "delimiter (\\t)"="," ("delimiter (\\t)")) -> ()  [unwired: 9 in, 2 out]
          }
        }
        n285 = stacked-sequence {
          tunnel: w502 -> [w509 _ _]
          tunnel: [_ _ 0] -> w501
          frame #0 {
            n286 = disable-structure shown="Enabled" {
              disable-tunnel: [w510 TRUE ("Tracibility")] -> w508
              frame Disabled {
                n287 = global read "Galobal variable_TI.vi" "Tracibility"() -> (w510:bool)
              }
              frame Enabled {
              }
            }
            n288 = case shown="True" w508 {
              tunnel: w509 -> [_ w515]
              frame False {
              }
              frame True {
                n289 = Increment(x=w515) -> (x+1=w514:i32)
                n290 = Number To Decimal String(number=w514) -> (decimal integer string=w516:string)  [unwired: 1 in]
                n291 = Bundle By Name(cluster=T8 {"No. Fail Coun t"="", "Rework Status Count 0\\1"="", "NA Count Max =3 "="", "Testesd Count  0/1"="", "Error code"=""} ("Count For Rework"), "No. Fail Coun t"=w516, "Rework Status Count 0\\1"="0" ("Rework Status Count 0\\1"), "NA Count Max =3"="0", "Testesd Count  0/1"="1") -> (w513:T8)
                n292 = call "Rework Count.vi"("Read /Write"=enum16{"Write", "Read"}."Write", "Count For Rework"=w513) -> ()  [unwired: 8 in, 2 out]
              }
            }
          }
          frame #1 {
            n293 = Wait (ms)(milliseconds to wait=u32 300) -> ()  [unwired: 1 out]
          }
          frame #2 {
            n294 = global write "Galobal variable_TI.vi" "Rpt Write"(TRUE ("Rpt Write")) -> ()
          }
        }
        n295 = call "Auotmode.vi"("Enum Selection"=Auot_Test_selection."Enqueue ", "Error In"=w505, "queue in"=w507) -> ("error out"=w504:errorcluster, "queue Out"=w506:refnum<queue>)  [unwired: 5 in, 1 out]
      }
      frame "Exit" {
        n296 = global read "Galobal variable_TI.vi" "Digital input"() -> (w575:bool[])
        n297 = stacked-sequence {
          tunnel: T9."LCD Rotation Up(P0.27_11)" ("Enum") -> [w581 _ _ _]
          frame #0 {
            n298 = call "Home Call Cylender.vi"("Enum"=w581) -> ()  [unwired: 11 in]
          }
          frame #1 {
            n299 = Wait (ms)(milliseconds to wait=u32 100) -> ()  [unwired: 1 out]
          }
          frame #2 {
            n300 = global read "Galobal variable_TI.vi" "Manual DO"() -> (w584:bool[])
            n301 = Replace Array Subset(array=w584, new element #1=FALSE ("new element/subarray"), index #1=13 ("index"), new element #2=TRUE ("new element/subarray"), index #2=14 ("index")) -> (w583:bool[])
            n302 = global write "Galobal variable_TI.vi" "Manual DO"(w583) -> ()
          }
          frame #3 {
            n303 = Wait (ms)(milliseconds to wait=u32 100) -> ()  [unwired: 1 out]
          }
        }
        n304 = Index Array(array=w575, index #1=30 ("index"), index #2=33 ("index"), index #3=2 ("index")) -> (element #1=w569:bool, element #2=w568:bool, element #3=w565:bool)
        n305 = global write "GR_Servo.vi" "Error Message"("Wait  LCD Display Unit _AI17") -> ()
        n306 = And(x=w569, y=w568) -> (x .and. y?=w567:bool)
        n307 = global write "GR_Servo.vi" "Error Color"(1 ("Error Color")) -> ()
        n308 = Select(t=AutoTest_seq."Poll Event" ("Enqueue"), s=w567, f=AutoTest_seq."Exit" ("Enqueue")) -> (s? t:f=w563:T2)
        n309 = Select(t=AutoTest_seq."Poll Event" ("Enqueue"), s=w565, f=w563) -> (s? t:f=w562:T2)
        n310 = call "Auotmode.vi"("Enum Selection"=Auot_Test_selection."Enqueue ", "Enqueue"=w562, "queue in"=w577) -> ("queue Out"=w578:refnum<queue>)  [unwired: 5 in, 2 out]
      }
    }
    n311 = global read "Galobal variable_TI.vi" "Auto Exit"() -> (w171:bool)
  }
  n312 = while {
    stop <- w591 stop-if-true
    n313 = event shown="[0] Timeout" {
      selector: _ -> [_ _ _ _]
      dyn-events: _ -> [_ _ _ _]
      timeout: 20 -> [_ _ _ _]
      event Timeout {
        (unwired) 9 ("index")
        w636 = cluster{u32, u32}[] [{16734762, 16711680}, {16777222, 16775560}] ("Colors [4]")
        w637 = cluster{u32, u32}[] [{16734762, 6618880}, {16777222, 6618880}] ("Colors [4]")
        n314 = event-data() -> ()  [unwired: 1 in, 3 out]
        n315 = call "H.Signal.vi"() -> ("H.Signal"=w621:T13, "Error Message"=w617:string)  [unwired: 10 in, 4 out]
        n316 = Unbundle By Name(w621) -> ("Emergency"=w610:bool, "Air Pressure"=w620:bool, "Saftey Sensor"=w619:bool, "Slide Servo  fault"=w593:bool, "LCD Pressing  Servo  fault"=w608:bool, "Reset"=w592:bool)
        n317 = global read "Galobal variable_TI.vi" "Digital input"() -> (w641:bool[])
        n318 = global read "GR_Servo.vi" "Error Color"() -> (w615:i32)
        n319 = global read "GR_Servo.vi" "Error Message"() -> (w618:string)
        n320 = Index Array(array=w641, index #1=26 ("index"), index #2=27 ("index"), index #3=18 ("index"), index #4=19 ("index"), index #5=12 ("index"), index #6=13 ("index")) -> (element #1=w602:bool, element #2=w600:bool, element #3=→"Difusser_AI4":bool, element #4=→"Difusser_AI5":bool)  [unwired: 2 out]
        n321 = Not(x=w620) -> (.not. x?=w609:bool)
        n322 = Index Array(array=w641, index #1=8 ("index"), index #2=9 ("index"), index #3=0 ("index"), index #4=3 ("index")) -> (element #1=w594:bool, element #2=w605:bool, element #3=→"Start":bool, element #4=→"Home":bool)
        n323 = Compound Arithmetic op=OR(w610, w609, w593, w608) -> (w606:bool)
        n324 = Compound Arithmetic op=OR(w610, w609, w619, w593, w608) -> (w607:bool)
        n325 = case shown="True" w592 {
          frame False {
          }
          frame True {
            n326 = global write "GR_Servo.vi" "Error Color"(0 ("y")) -> ()
          }
        }
        n327 = global read "Galobal variable_TI.vi" "STM Done Bit"() -> (w647:bool)
        n328 = Select(t=w617, s=w606, f=w618) -> (s? t:f=w616:string)
        n329 = Select(t=1 ("y"), s=w606, f=w615) -> (s? t:f=w613:i32)
        n330 = Not(x=w602) -> (.not. x?=w601:bool)
        n331 = Equal?(x=w613, y=0) -> (x = y?=w630:bool)
        n332 = global read "GR_Servo.vi" "Error Color"() -> (w624:i32)
        n333 = Or(x=w594, y=w647) -> ()  [unwired: 1 out]
        n334 = global write "Galobal variable_TI.vi" "Stop M1"(w607) -> ()
        n335 = global write "Galobal variable_TI.vi" "Stop M2"(w607) -> ()
        n336 = local read "Cycle Start Bit"() -> (w611:bool)
        n337 = Not(x=w605) -> (.not. x?=w595:bool)
        n338 = Equal?(x=w624, y=1) -> (x = y?=w626:bool)
        n339 = Compound Arithmetic op=OR(w601, w600, w595) -> (w599:bool)
        n340 = Select(t=u32 16777226 ("Color Box"), s=w630, f=u32 16711680 ("Color Box")) -> (s? t:f=w627:u32)
        n341 = Select(t=u32 16777226 ("Color Box"), s=w626, f=u32 16711680 ("Color Box")) -> ()  [unwired: 1 out]
        n342 = Select(t=enum32{"Image Display", "Load Graph"}."Load Graph" ("Tab"), s=w599, f=enum32{"Image Display", "Load Graph"}."Image Display" ("Tab")) -> (s? t:f=w596:enum32{"Image Display", "Load Graph"})
        n343 = case shown="False" w611 {
          tunnel: w606 -> [w652 _]
          tunnel: w593 -> [w651 _]
          tunnel: w592 -> [w650 _]
          frame False {
            n344 = case shown="True" w651 {
              tunnel: w652 -> [w653 _]
              tunnel: w650 -> [_ w662]
              frame False {
                n345 = case shown="False" w653 {
                  frame False {
                    n346 = call "Tower light.vi"("Enum"=enum16{"Green", "Red", "Yellow", "OFF"}."Yellow") -> ()  [unwired: 11 in]
                  }
                  frame True {
                    n347 = call "Tower light.vi"("Enum"=enum16{"Green", "Red", "Yellow", "OFF"}."Red") -> ()  [unwired: 11 in]
                  }
                }
              }
              frame True {
                n348 = global read "Galobal variable_TI.vi" "Manual DO"() -> (w659:bool[])
                n349 = Select(t=TRUE, s=w662, f=FALSE) -> (s? t:f=w658:bool)
                n350 = Replace Array Subset(array=w659, new element=w658, index=1) -> (w656:bool[])
                n351 = global write "Galobal variable_TI.vi" "Manual DO"(w656) -> ()
              }
            }
          }
          frame True {
          }
        }
        n352 = Select(t=w637, s=w594, f=w636) -> (s? t:f=w648:cluster{u32, u32}[])
        n353 = Select(t=w637, s=w605, f=w636) -> (s? t:f=w635:cluster{u32, u32}[])
        n354 = property on="Error Message" class="Str"("Value"=w616, "Text.BGColor"=w627) -> ()  [unwired: 2 in, 2 out]
        n355 = local write "Tab"(w596) -> ()
        n356 = property on="Slide Servo Home Call" class="Bool (strict)"("Colors [4]"=w648) -> ()  [unwired: 2 in, 2 out]
        n357 = property on="LCD Servo Call" class="Bool (strict)"("Colors [4]"=w635) -> ()  [unwired: 2 in, 2 out]
      }
      event "Home": Value Change {
        n358 = event-data() -> ()  [unwired: 1 in, 6 out]
        n359 = local write "Tab Control"(enum32{"Test", "Home call"}."Home call" ("Tab Control")) -> ()
      }
      event "Start": Value Change {
        n360 = event-data() -> ()  [unwired: 1 in, 6 out]
        n361 = local write "Tab Control"(enum32{"Test", "Home call"}."Test" ("Tab Control")) -> ()
      }
      event Value Change {
        n362 = event-data() -> ("NewVal"=w665:T4)  [unwired: 1 in]
        n363 = global read "Galobal variable_TI.vi" "Digital input"() -> (→"DI":bool[])
        n364 = global write "Galobal variable_TI.vi" "Auto Exit"(w665) -> ()
      }
    }
    n365 = local read "Exit"() -> (w591:T4)
  }
  n366 = call "Auotmode.vi"("Enum Selection"=Auot_Test_selection."Flush", "Error In"=w50, "queue in"=w57) -> ("error out"=w62:errorcluster, "queue Out"=w61:refnum<queue>)  [unwired: 5 in, 1 out]
  n367 = call "Auotmode.vi"("Enum Selection"=Auot_Test_selection."Release Queue", "Error In"=w62, "queue in"=w61) -> ("error out"=→"error out":errorcluster)  [unwired: 5 in, 2 out]
